vi "$CTL_LevelCtlr.vi"(6 "error in (no error)":errorcluster={"status"=TRUE, "code"=524288, "source"="eyence LK-G3000.lvlib:LKIF_GetCalcData.vi"}, 7 "VISA Refnum in":refnum<visa-resource-name>, 8 "Pump Params":T3={"Empty Inches"=8.4, "Full Inches"=2.6, "RNG_SLOW"=0.5, "RNG_CREEP"=0.007, "RNG_STOP "=0.002, "VISA resource name"="Default", "SPD_SLOW"=30, "SPD_CREEP"=7, "SPD_FAST"=100, "Zero template"=path "30", "zero  Settle sec"=5, "Laser Slope"=-0.996, "Laser Offset"=9.601, "Sim Fill Rate"=2000.0, "Cal Date"="CAL_Level_RnR_241105.xlsx", "Cal Technician"="7"} {"Sim Fill Rate" format="%.3f"; "Laser Offset" format="%.3f"; "Laser Slope" format="%.3f"; "RNG_STOP" format="%#_13g"; "RNG_CREEP" format="%#_13g"; "RNG_SLOW" format="%#_13g"}, 9 "Pump Manual Controls":T4={"Pump Speed"=enum."STOP", "FILL"=FALSE, "Drain"=FALSE, "Auto/!Man"=TRUE, "Sim Level"=TRUE, "Raw Leve/\n!Level PVl"=FALSE, "Jog"=TRUE}, 10 "Level SP":dbl(slide)=8.4 scale=0.0..10.0) -> (0 "Pump Speed Out":T2=enum."STOP", 1 "Level Out":T1={"Laser "={"Raw"=0.0, "Scaled"=9.60099983215332}, "Level PV"=9.60099983215332, "Fill"=FALSE, "Drain"=FALSE}, 2 "Auto/!Man":bool=TRUE, 3 "Pump On Line":bool=TRUE, 4 "error out":errorcluster, 5 "VISA Refnum out":refnum<visa-resource-name>)   [LabVIEW 2024]
uses:
  Control Definitions/DEF_PumpManCtl.ctl
  Control Definitions/Def_PumpSpeed.ctl
  Control Definitions/DEF_PumpParams.ctl
  Control Definitions/DEF_LevelOut.ctl
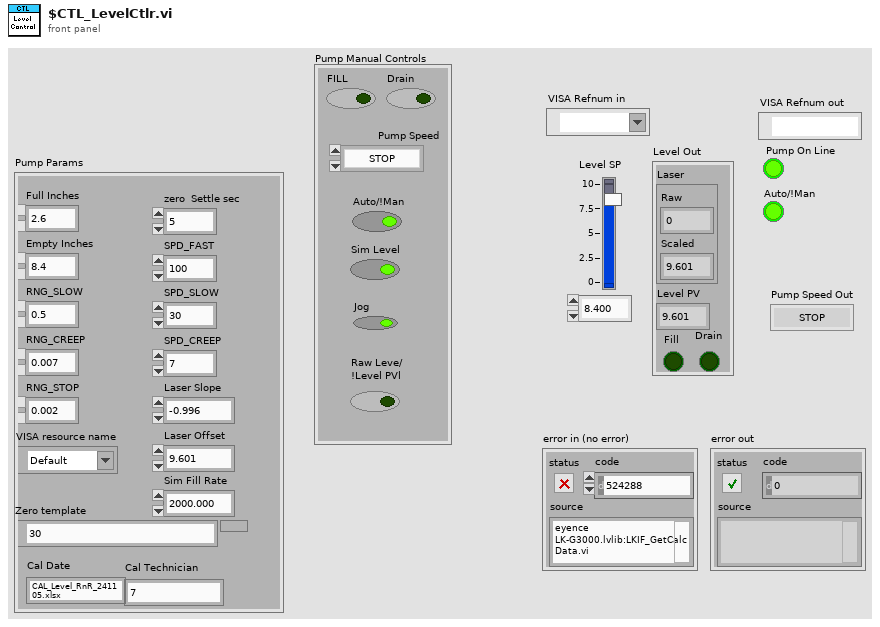
[diagram p1: front panel]
types:
  T1 = typedef "DEF_LevelOut.ctl" = cluster{"Laser ":cluster{"Raw":sgl, "Scaled":dbl}, "Level PV":dbl, "Fill":bool, "Drain":bool}
  T2 = typedef "Def_PumpSpeed.ctl" = enum16{"FAST", "SLOW", "CREEP", "STOP"}
  T3 = typedef "DEF_PumpParams.ctl" = cluster{"Empty Inches":dbl, "Full Inches":dbl, "RNG_SLOW":dbl, "RNG_CREEP":dbl, "RNG_STOP ":dbl, "VISA resource name":refnum<visa-resource-name>, "SPD_SLOW":i32, "SPD_CREEP":i32, "SPD_FAST":i32, "Zero template":path, "zero  Settle sec":i32, "Laser Slope":sgl, "Laser Offset":sgl, "Sim Fill Rate":sgl, "Cal Date":string, "Cal Technician":string}
  T4 = typedef "DEF_PumpManCtl.ctl" = cluster{"Pump Speed":T2, "FILL":bool, "Drain":bool, "Auto/!Man":bool, "Sim Level":bool, "Raw Leve/\n!Level PVl":bool, "Jog":bool}
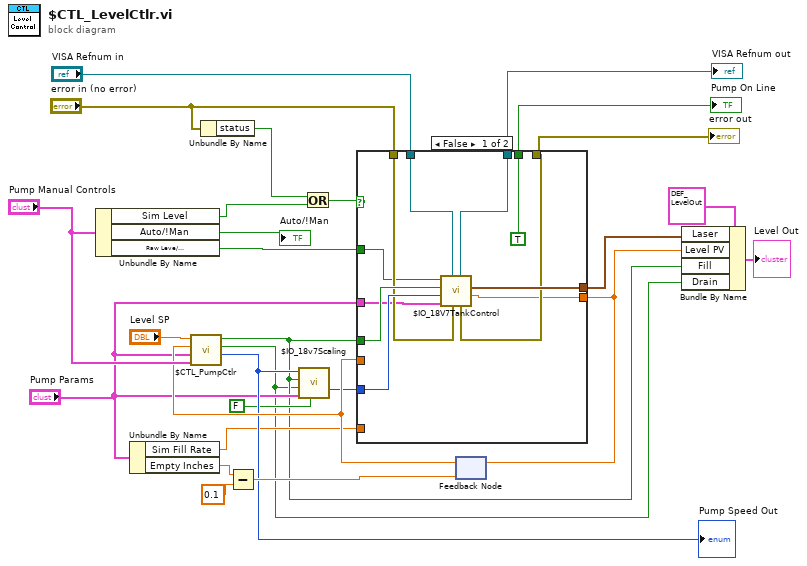
[diagram p0: block diagram]
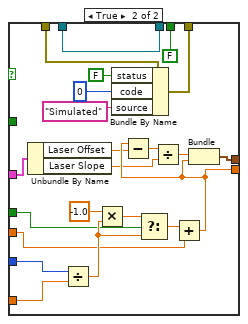
[diagram p2: hidden frame]
diagram:
  n1 = Unbundle By Name("Pump Manual Controls") -> ("Sim Level"=w11:bool, "Auto/!Man"=→"Auto/!Man":bool, "Raw Leve/\n!Level PVl"=w10:bool)
  n2 = Unbundle By Name("Pump Params") -> ("Sim Fill Rate"=w7:sgl, "Empty Inches"=w22:dbl)
  n3 = Unbundle By Name("error in (no error)") -> ("status"=w1:bool)
  n4 = Subtract(x=w22, y=0.1) -> (x-y=w24:dbl)
  n5 = Or(x=w1, y=w11) -> (x .or. y?=w26:bool)
  n6 = feedback #1(w24) -> (w23:dbl)
  n7 = call "$CTL_PumpCtlr.vi"("Pump Manual Controls"="Pump Manual Controls", "Pump Params"="Pump Params", "Level PV"=w23, "Level SP"="Level SP") -> ("Pump Speed Out"=w16:T2, "X< Neg"=w2:bool, "X>Pos"=w3:bool)  [unwired: 4 in, 1 out]
  "Pump Speed Out" <- w16
  n8 = call "$IO_18v7Scaling.vi"("!Enabled"=FALSE, "Pump Params"="Pump Params", "Drain"=w2, "Fill"=w3, "Pump Speed"=w16) -> ("Speed Out"=w17:i32)  [unwired: 5 in, 1 out]
  n9 = case shown="False" w26 {
    tunnel: w23 -> [_ w52]
    tunnel: [w38 w42] -> w9
    tunnel: w3 -> [w37 w53]
    tunnel: w17 -> [w36 w56]
    tunnel: [w31 w57] -> w14
    tunnel: [w33 w47] -> w18
    tunnel: "VISA Refnum in" -> [w32 w57]
    tunnel: "error in (no error)" -> [w34 w51]
    tunnel: [TRUE FALSE] -> w19
    tunnel: w10 -> [w29 _]
    tunnel: [w30 w43] -> w8
    tunnel: w7 -> [_ w46]
    tunnel: "Pump Params" -> [w28 w39]
    frame False {
      n10 = call "$IO_18V7TankControl.vi"("error in"=w34, "VISA Refnum in"=w32, "Pump Params"=w28, "Speed"=w36, "Fill!Drain"=w37, "Raw/!Saled Level"=w29) -> ("Level PV"=w30:sgl, "Level"=w38:cluster{"Laser Raw":sgl, "Laser Scaled":dbl}, "error out"=w33:errorcluster, "VISA Refnum out"=w31:refnum<visa-resource-name>)  [unwired: 2 in]
    }
    frame True {
      n11 = Unbundle By Name(w39) -> ("Laser Offset"=w40:sgl, "Laser Slope"=w41:sgl)
      n12 = Divide(x=w56, y=w46) -> (x/y=w59:sgl)
      n13 = Multiply(x=-1.0 ("y"), y=w59) -> (x*y=w60:dbl)
      n14 = Bundle By Name(cluster=w51, "status"=FALSE, "code"=0, "source"="Simulated") -> (w47:errorcluster)
      n15 = Select(t=w60, s=w53, f=w59) -> (s? t:f=w55:dbl)
      n16 = Add(x=w55, y=w52) -> (x+y=w43:dbl)
      n17 = Subtract(x=w43, y=w40) -> (x-y=w45:dbl)
      n18 = Divide(x=w45, y=w41) -> (x/y=w44:dbl)
      n19 = Bundle(w44, w43) -> (w42:cluster{dbl, dbl})  [unwired: 1 in]
    }
  }
  "Pump On Line" <- w19
  "error out" <- w18
  "VISA Refnum out" <- w14
  n20 = feedback-in #1(w8) -> ()
  n21 = Bundle By Name(cluster=T1 {"Laser "={"Raw"=4.12249, "Scaled"=5.494999983534218}, "Level PV"=5.494999983534218, "Fill"=FALSE, "Drain"=FALSE} ("Level Out"), "Laser"=w9, "Level PV"=w8, "Fill"=w3, "Drain"=w2) -> (→"Level Out":T1)
